vi "4 Axis - Enable.vi"(4 "error in (no error)":errorcluster, 5 "Enable/Disable":bool=TRUE, 7 "Controller Reference":refnum<k7>) -> (0 "error out":errorcluster, 3 "Controller Reference out":refnum<k7>)   [LabVIEW 2015]
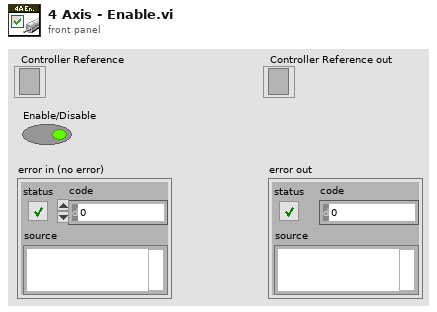
[diagram p1: front panel]
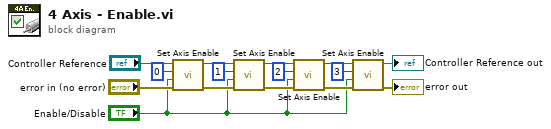
[diagram p0: block diagram]
diagram:
  n1 = call "Set Axis Enable.vi"("error in (no error)"="error in (no error)", "Enable/Disable"="Enable/Disable", "Axis In"=i16 0, "Controller Reference"="Controller Reference") -> ("error out"=w11:errorcluster, "Controller Reference out"=w12:refnum<k7>)  [unwired: 1 in, 1 out]
  n2 = call "Set Axis Enable.vi"("error in (no error)"=w11, "Enable/Disable"="Enable/Disable", "Axis In"=i16 1, "Controller Reference"=w12) -> ("error out"=w8:errorcluster, "Controller Reference out"=w9:refnum<k7>)  [unwired: 1 in, 1 out]
  n3 = call "Set Axis Enable.vi"("error in (no error)"=w8, "Enable/Disable"="Enable/Disable", "Axis In"=i16 2, "Controller Reference"=w9) -> ("error out"=w5:errorcluster, "Controller Reference out"=w6:refnum<k7>)  [unwired: 1 in, 1 out]
  n4 = call "Set Axis Enable.vi"("error in (no error)"=w5, "Enable/Disable"="Enable/Disable", "Axis In"=i16 3, "Controller Reference"=w6) -> ("error out"=→"error out":errorcluster, "Controller Reference out"=→"Controller Reference out":refnum<k7>)  [unwired: 1 in, 1 out]
